vi "TC_alarm_to_array.vi"(11 "TC_alarms":T1[](array[typedef])) -> (1 "TC_channel_data":dbl[][](array[numeric]), 2 "TimeStamp":dbl[](array[numeric]), 3 "TimeString":string[](array[string]))   [LabVIEW 2018]
doc: "Timestamp, timestring and corresponding TC_alarm datapoint for each TC_alarm channel."
uses:
  HDF5/TC_Data_Structure.ctl
panel:
  # "Channels in columns\nTimestamp row correpsonds to datapoint in channel data row"
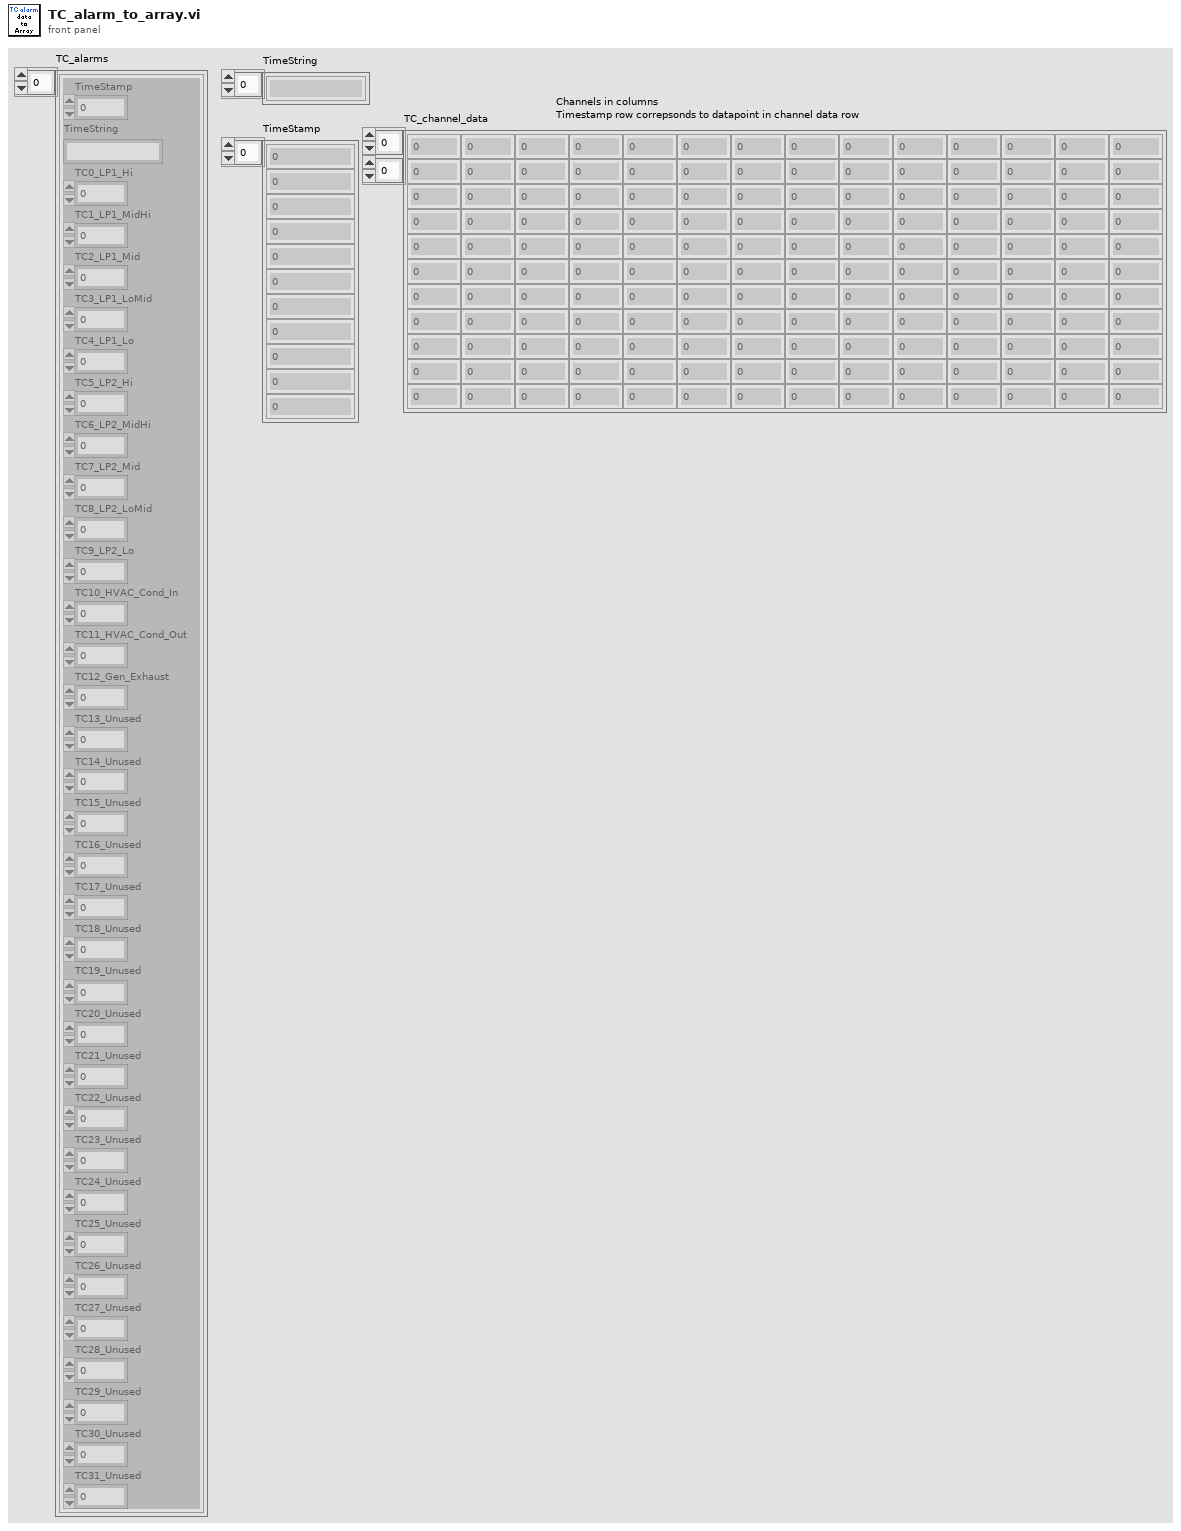
[diagram p1: front panel]
types:
  T1 = typedef "TC_Data_Structure.ctl" = cluster{"TimeStamp":dbl, "TimeString":string, "TC0_LP1_Hi":dbl, "TC1_LP1_MidHi":dbl, "TC2_LP1_Mid":dbl, "TC3_LP1_LoMid":dbl, "TC4_LP1_Lo":dbl, "TC5_LP2_Hi":dbl, "TC6_LP2_MidHi":dbl, "TC7_LP2_Mid":dbl, "TC8_LP2_LoMid":dbl, "TC9_LP2_Lo":dbl, "TC10_HVAC_Cond_In":dbl, "TC11_HVAC_Cond_Out":dbl, "TC12_Gen_Exhaust":dbl, "TC13_Unused":dbl, "TC14_Unused":dbl, "TC15_Unused":dbl, "TC16_Unused":dbl, "TC17_Unused":dbl, "TC18_Unused":dbl, "TC19_Unused":dbl, "TC20_Unused":dbl, "TC21_Unused":dbl, "TC22_Unused":dbl, "TC23_Unused":dbl, "TC24_Unused":dbl, "TC25_Unused":dbl, "TC26_Unused":dbl, "TC27_Unused":dbl, "TC28_Unused":dbl, "TC29_Unused":dbl, "TC30_Unused":dbl, "TC31_Unused":dbl}
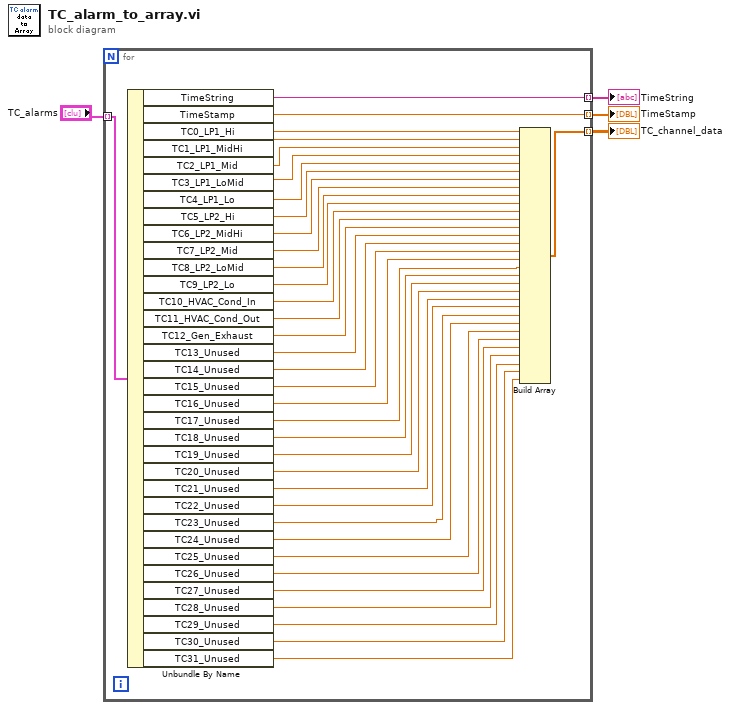
[diagram p0: block diagram]
diagram:
  n1 = for {
    tunnel: "TC_alarms" -> [w40] mode=indexing
    tunnel: [w39] -> w3 mode=indexing
    tunnel: [w38] -> w2 mode=indexing
    tunnel: [w36] -> w4 mode=indexing
    n2 = Unbundle By Name(w40) -> ("TimeString"=w39:string, "TimeStamp"=w38:dbl, "TC0_LP1_Hi"=w37:dbl, "TC1_LP1_MidHi"=w35:dbl, "TC2_LP1_Mid"=w34:dbl, "TC3_LP1_LoMid"=w33:dbl, "TC4_LP1_Lo"=w32:dbl, "TC5_LP2_Hi"=w31:dbl, "TC6_LP2_MidHi"=w30:dbl, "TC7_LP2_Mid"=w29:dbl, "TC8_LP2_LoMid"=w28:dbl, "TC9_LP2_Lo"=w27:dbl, "TC10_HVAC_Cond_In"=w26:dbl, "TC11_HVAC_Cond_Out"=w25:dbl, "TC12_Gen_Exhaust"=w24:dbl, "TC13_Unused"=w23:dbl, "TC14_Unused"=w22:dbl, "TC15_Unused"=w21:dbl, "TC16_Unused"=w20:dbl, "TC17_Unused"=w19:dbl, "TC18_Unused"=w18:dbl, "TC19_Unused"=w17:dbl, "TC20_Unused"=w16:dbl, "TC21_Unused"=w15:dbl, "TC22_Unused"=w14:dbl, "TC23_Unused"=w13:dbl, "TC24_Unused"=w12:dbl, "TC25_Unused"=w11:dbl, "TC26_Unused"=w10:dbl, "TC27_Unused"=w9:dbl, "TC28_Unused"=w8:dbl, "TC29_Unused"=w7:dbl, "TC30_Unused"=w6:dbl, "TC31_Unused"=w5:dbl)
    n3 = Build Array(w37, w35, w34, w33, w32, w31, w30, w29, w28, w27, w26, w25, w24, w23, w22, w21, w20, w19, w18, w17, w16, w15, w14, w13, w12, w11, w10, w9, w8, w7, w6, w5) -> (w36:dbl[])
  }
  "TC_channel_data" <- w4
  "TimeString" <- w3
  "TimeStamp" <- w2
